vi "String Contains Quote(s).vi"(2 "String":string) -> (7 "Contains quotes?":bool)   [LabVIEW 2021, in "Strings.lvlib"]
uses:
  Strings.lvlib
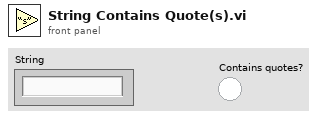
[diagram p1: front panel]
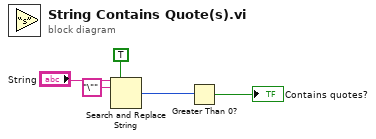
[diagram p0: block diagram]
diagram:
  n1 = Search and Replace String(replace all?=TRUE ("replace all? (F)"), input string="String", search string="\"") -> (number of replacements=w2:i32)  [unwired: 5 in, 3 out]
  n2 = Greater Than 0?(x=w2) -> (x > 0?=→"Contains quotes?":bool)
